vi "Rotate.vi"(8 "error in (no error)":errorcluster, 10 "Angle (deg)":dbl, 11 "Point in":refnum<class "PointSpecialized.lvclass">) -> (0 "error out":errorcluster, 3 "Point out":refnum<class "PointSpecialized.lvclass">)   [LabVIEW 2021, in "Picture2D.lvlib" / "PointSpecialized.lvclass"]
uses:
  PointSpecialized.lvclass
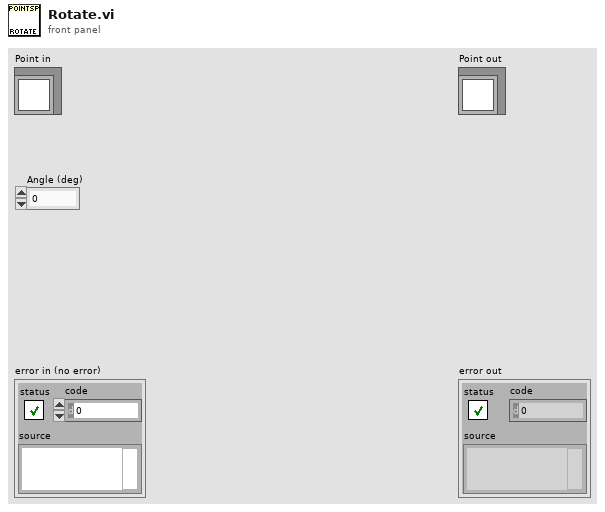
[diagram p1: front panel]
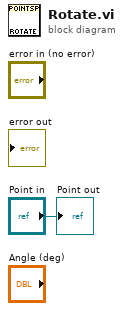
[diagram p0: block diagram]
diagram:
  "Point out" <- "Point in"
